vi "GOOP_VI_Provider_OnPopupMenu.vi"(11 "objects":T1[](array[typedef])) -> ()   [LabVIEW 2020]
uses:
  <resource>/Framework/Providers/API/ItemRef.ctl
  <resource>/Framework/Providers/API/mxLvMenuItem.ctl
panel:
  out "error out":errorcluster
  in  "error in":errorcluster
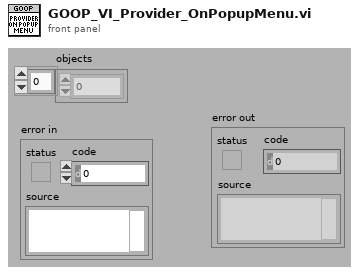
[diagram p1: front panel]
types:
  T1 = typedef "ItemRef.ctl" = u64
  T2 = typedef "mxLvMenuItem.ctl" = cluster{"Menu Name":string, "Description":string, "Icon File Name":path, "Menu Tag":string, "Enabled":bool, "Checked":bool, "Separator":bool, "Batchable":bool, "Weight":i32, "Batch Mode (Ignored if Not Batchable)":enum32{"Show If All Items Support Command", "Show If Any Items Support Command"}, "Menu Location":enum32{"<None>", "Project", "Project / Build Specifications", "Tools", "Tools / Source Control", "Tools / Real-Time Module", "Help"}, "Exclude From Getting Started Window Menu":bool}
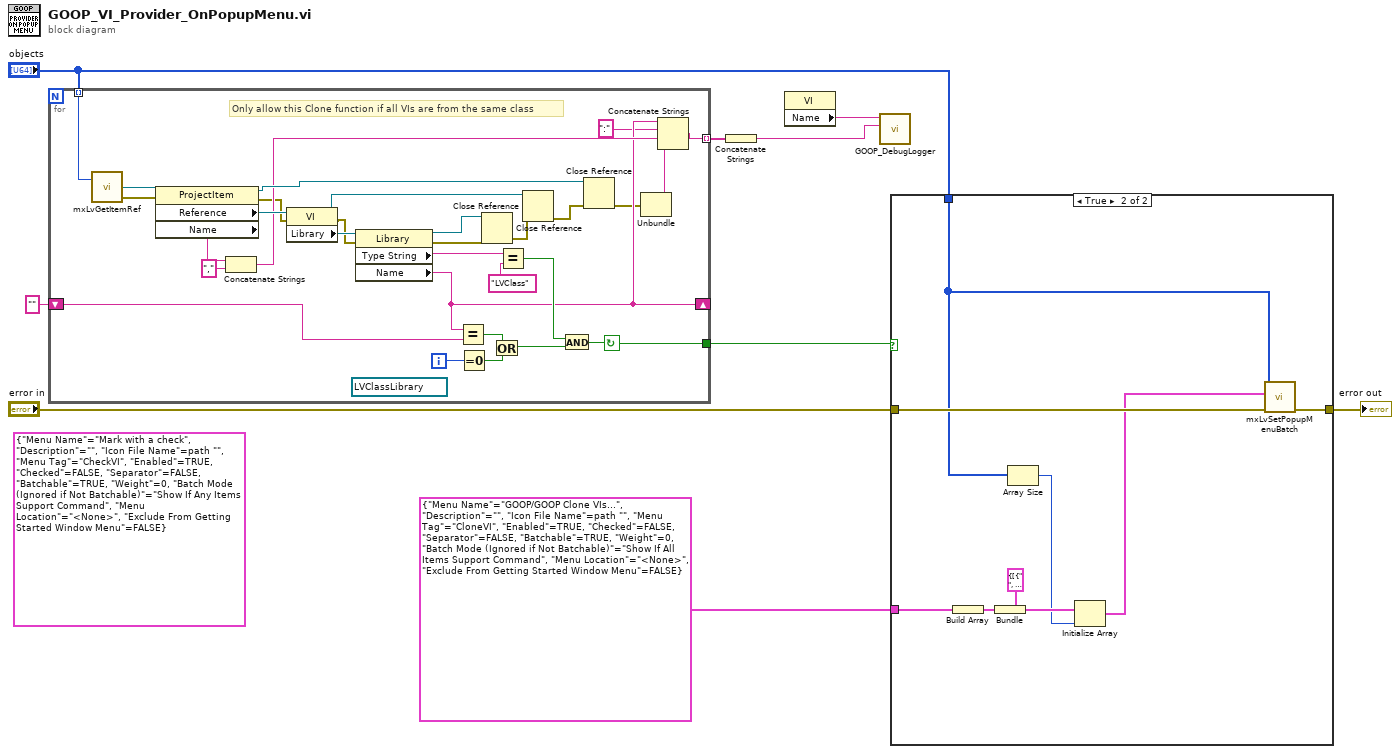
[diagram p0: block diagram]
diagram:
  (unwired) T2 {"Menu Name"="Mark with a check", "Description"="", "Icon File Name"=path "", "Menu Tag"="CheckVI", "Enabled"=TRUE, "Checked"=FALSE, "Separator"=FALSE, "Batchable"=TRUE, "Weight"=0, "Batch Mode (Ignored if Not Batchable)"=enum."Show If Any Items Support Command", "Menu Location"=enum."<None>", "Exclude From Getting Started Window Menu"=FALSE} ("Menu Item")
  n1 = for {
    tunnel: "objects" -> [w39] mode=indexing
    shift-right: [w17] -> _
    shift-left: "" ("Name") -> [w27]
    tunnel: [w21] -> w4
    tunnel: [w16] -> w2 mode=indexing
    i -> [w26]
    stop <- w21 continue-if-true
    (unwired) refnum<vi> refnum ("Library")
    # "Only allow this Clone function if all VIs are from the same class"
    n2 = call <resource>:"mxLvGetItemRef.vi"("Item"=w39) -> ("Item Refnum"=w38:refnum<vi>, "error out"=w10:errorcluster)  [unwired: 1 in, 1 out]
    n3 = property class="ProjectItem"(reference=w38, error in=w10) -> (reference out=w28:refnum<vi>, error out=w11:errorcluster, "Reference"=w37:refnum<vi>, "Name"=w20:string)
    n4 = Concatenate Strings(w20, "," ("string")) -> (w18:string)
    n5 = property class="VI"(reference=w37, error in=w11) -> (reference out=w31:refnum<vi>, error out=w12:errorcluster, "Library"=w36:refnum<vi>)
    n6 = property class="Library"(reference=w36, error in=w12) -> (reference out=w32:refnum<vi>, error out=w33:errorcluster, "Type String"=w35:string, "Name"=w17:string)
    n7 = Equal?(x=w17, y=w27) -> (x = y?=w25:bool)
    n8 = Equal To 0?(x=w26) -> (x = 0?=w24:bool)
    n9 = Close Reference(reference=w32, error in (no error)=w33) -> (error out=w30:errorcluster)
    n10 = Or(x=w25, y=w24) -> (x .or. y?=w23:bool)
    n11 = Equal?(x=w35, y="LVClass") -> (x = y?=w22:bool)
    n12 = Close Reference(reference=w31, error in (no error)=w30) -> (error out=w29:errorcluster)
    n13 = And(x=w22, y=w23) -> (x .and. y?=w21:bool)
    n14 = Close Reference(reference=w28, error in (no error)=w29) -> (error out=w14:errorcluster)
    n15 = Unbundle(w14) -> ("source"=w13:string)  [unwired: 2 out]
    n16 = Concatenate Strings(w17, ":", w18, w13) -> (w16:string)
  }
  n17 = Concatenate Strings(w2) -> (w1:string)
  n18 = property class="VI"() -> ("Name"=w3:string)  [unwired: 2 in, 2 out]
  n19 = call <resource>:"GOOP_DebugLogger.vi"("Data"=w1, "State"=w3) -> ()  [unwired: 7 in, 3 out]
  n20 = case shown="True" w4 {
    tunnel: [w40 w49] -> w9
    tunnel: "error in" -> [w40 w48]
    tunnel: T2 {"Menu Name"="GOOP/GOOP Clone VIs...", "Description"="", "Icon File Name"=path "", "Menu Tag"="CloneVI", "Enabled"=TRUE, "Checked"=FALSE, "Separator"=FALSE, "Batchable"=TRUE, "Weight"=0, "Batch Mode (Ignored if Not Batchable)"=enum."Show If All Items Support Command", "Menu Location"=enum."<None>", "Exclude From Getting Started Window Menu"=FALSE} ("Menu Item") -> [_ w46]
    tunnel: "objects" -> [_ w42]
    frame False {
    }
    frame True {
      n21 = Build Array(w46) -> (w45:T2[])
      n22 = Bundle(cluster=cluster{"Popup Menu Items":T2[]} {"Popup Menu Items"=[{"Menu Name"="", "Description"="", "Icon File Name"=path "", "Menu Tag"="", "Enabled"=TRUE, "Checked"=FALSE, "Separator"=FALSE, "Batchable"=TRUE, "Weight"=0, "Batch Mode (Ignored if Not Batchable)"=enum."Show If Any Items Support Command", "Menu Location"=enum."<None>", "Exclude From Getting Started Window Menu"=FALSE}]}, "Popup Menu Items"=w45) -> (w44:cluster{"Popup Menu Items":T2[]})
      n23 = Array Size(array=w42) -> (size(s)=w43:i32)
      n24 = Initialize Array(w44, w43) -> (w41:cluster{"Popup Menu Items":T2[]}[])
      n25 = call <resource>:"mxLvSetPopupMenuBatch.vi"("error in"=w48, "Menu Items"=w41, "Items"=w42) -> ("error out"=w49:errorcluster)  [unwired: 7 in, 1 out]
    }
  }
  "error out" <- w9
